vi "Launch Chronometer.vi"(8 "error in":errorcluster, 11 "Base Software in":refnum<class "Main.lvclass">) -> (0 "error out":errorcluster, 3 "Base Software out":refnum<class "Main.lvclass">)   [LabVIEW 2023, in "Main.lvlib" / "Main.lvclass"]
uses:
  Project/Main.lvclass
  C:/Users/Public/Documents/Development/builds/Engine/Engine.lvlibp/Project/Engine.lvclass
  builds/Engine/Panel Manager.lvlibp/Panel Actor/Panel Actor.lvclass
  builds/Engine/Panel.lvlibp/Panel/Panel.lvclass
  Custom Controls/Panel_Positions.ctl
  builds/Tools/Chronometer.lvlibp/Library/Chronometer.lvclass
  C:/Users/Public/Documents/Development/builds/Engine/Actor Framework.lvlibp/1abvi3w/vi.lib/ActorFramework/Actor/Actor.lvclass
  C:/Users/Public/Documents/Development/builds/Engine/Panel Manager.lvlibp/Panel Actor/Panel Actor.lvclass
  builds/Engine/Panel.lvlibp/Panel/Subpanel/Subpanel.lvclass
  C:/Users/Public/Documents/Development/builds/Engine/Panel.lvlibp/Panel/Panel.lvclass
  builds/Engine/Engine.lvlibp/Accessors/Read Directory.vi
  builds/Engine/Engine.lvlibp/Accessors/Read Events.vi
  Accessors/Indicators/Read Powered Time Ref.vi
  Accessors/GUI/Read Left Panel ref.vi
  builds/Engine/Panel.lvlibp/Panel/Subpanel/Subpanel.vi
  Custom Controls/g_Identifiers.vi
  builds/Engine/Actor Framework.lvlibp/1abvi3w/vi.lib/ActorFramework/Actor/Write Actor Label.vi
  builds/Engine/Engine.lvlibp/Accessors/Write Directory.vi
  builds/Engine/Engine.lvlibp/Accessors/Write Events.vi
  builds/Tools/Chronometer.lvlibp/Library/Accessors/Write Run_Time.vi
  builds/Engine/Panel.lvlibp
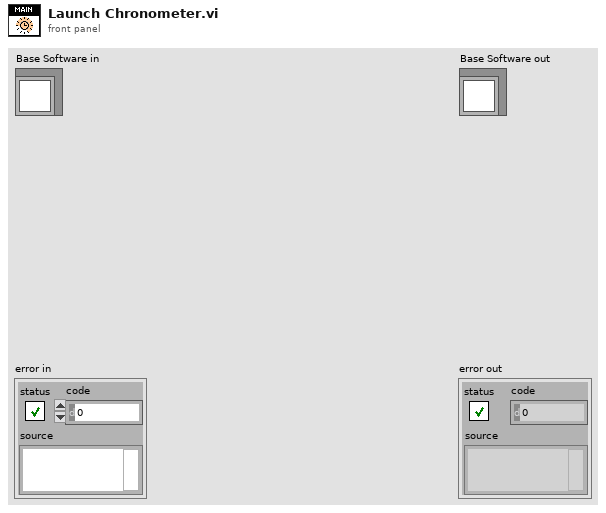
[diagram p1: front panel]
types:
  T1 = typedef "Main.lvlib/Main.lvclass/Panel_Positions.ctl" = enum16{"Prime", "Right", "Bottom", "Left", "Mission"}
  T2 = cluster{"Panel Actor":refnum<class "Panel Actor.lvclass">, "Panel":refnum<class "Panel.lvclass">}
  T3 = typedef "Engine.lvlibp/Engine.lvclass/Engine Events.ctl" = cluster{"System Event":T4, "Manual":T5, "UUT":T6, "Interface Events":T7}
  T4 = typedef "Engine.lvlibp/Engine.lvclass/System Events.ctl" = cluster{"Fault Event":refnum<user-event>, "SystemStatus Event":refnum<user-event>, "Automation":refnum<user-event>}
  T5 = typedef "Engine.lvlibp/Engine.lvclass/Manual Events.ctl" = cluster{"QuickStart Event":refnum<user-event>, "SafeBTE Event":refnum<user-event>, "TogglePower Event":refnum<user-event>, "Change Instrument Event":refnum<user-event>, "Toggle Launch Event":refnum<user-event>, "UUTSupply":refnum<user-event>}
  T6 = typedef "Engine.lvlibp/Engine.lvclass/UUT_Events.ctl" = cluster{"UUT_Name":refnum<user-event>, "Test_Name":refnum<user-event>, "Test_Operator":refnum<user-event>, "Test_Witness":refnum<user-event>, "Pedigree_Event":refnum<user-event>}
  T7 = typedef "Engine.lvlibp/Engine.lvclass/Interface Events.ctl" = cluster{"Interface_Command":refnum<user-event>, "Telemetry_Descriptor":refnum<user-event>, "AsynchTLM_Descriptor":refnum<user-event>}
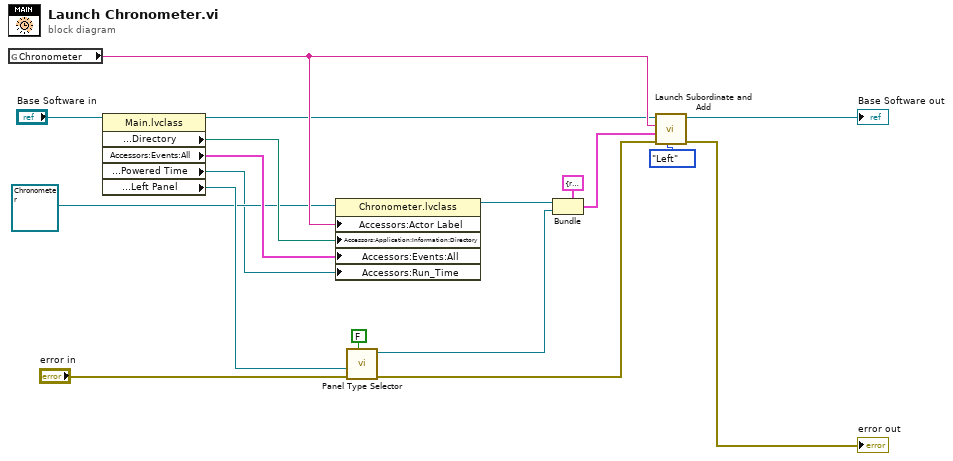
[diagram p0: block diagram]
diagram:
  n1 = global read "g_Identifiers.vi" "Chronometer"() -> (w17:string)
  n2 = property class="Main.lvclass"(reference="Base Software in") -> (reference out=w6:refnum<class "Main.lvclass">, "Accessors:Application:Information:Directory"=w4:path, "Accessors:Events:All"=w5:T3, "Accessors:Indicators:Powered Time"=w1:refnum<vi>, "Accessors:GUI:Panel_Pos:Left Panel"=w7:refnum<vi>)  [unwired: 1 in, 1 out]
  n3 = property class="Chronometer.lvclass"(reference=refnum<class "Chronometer.lvclass"> refnum ("Chronometer.lvlibp:Chronometer.lvclass"), "Accessors:Actor Label"=w17, "Accessors:Application:Information:Directory"=w4, "Accessors:Events:All"=w5, "Accessors:Run_Time"=w1) -> (reference out=w16:refnum<class "Chronometer.lvclass">)  [unwired: 1 in, 1 out]
  n4 = call-poly "Panel Type Selector.vi"("Autoshow? (T)"=FALSE, "Error In"="error in", "Sub Panel"=w7) -> ("Error Out"=w11:errorcluster, "Subpanel Out"=w13:refnum<class "Subpanel.lvclass">)  [unwired: 7 in]
  n5 = Bundle(cluster=T2 {"Panel Actor"=refnum, "Panel"=refnum} ("Panel Definiton"), "Panel Actor"=w16, "Panel"=w13) -> (w12:T2)
  n6 = call "Launch Subordinate and Add.vi"("Position"=Panel_Positions."Left", "error in"=w11, "Panel Definiton"=w12, "Identifier"=w17, "Base Software in"=w6) -> ("error out"=→"error out":errorcluster, "Base Software out"=→"Base Software out":refnum<class "Main.lvclass">)  [unwired: 5 in]
